vi "set_input_ref.vi"(8 "error in (no error)":errorcluster, 10 "input_ref":refnum<data-value>, 11 "input_poller in":refnum<class "input_poller.lvclass">) -> (0 "error out":errorcluster, 3 "input_poller out":refnum<class "input_poller.lvclass">)   [LabVIEW 2015, in "input_poller.lvclass"]
uses:
  input_poller.lvclass
  input.lvclass
  input_poller.lvclass/input_poller.ctl
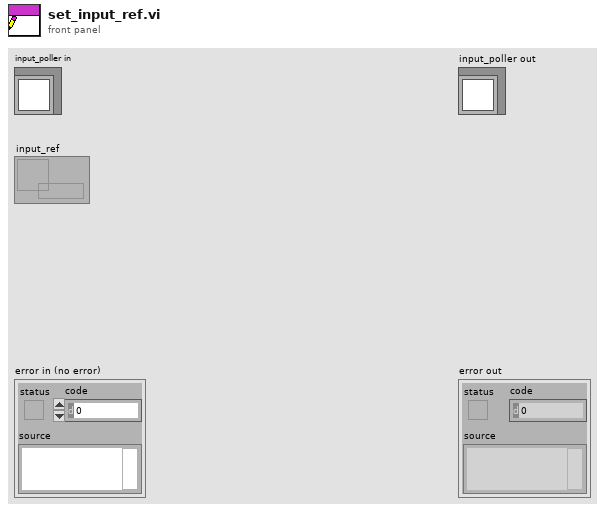
[diagram p1: front panel]
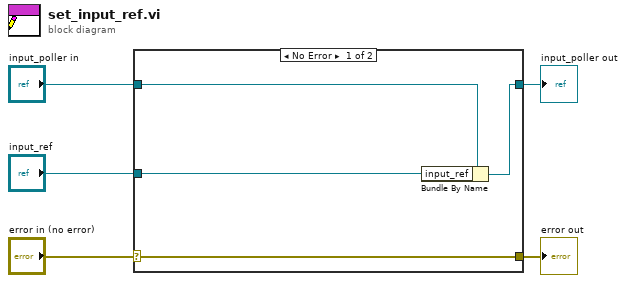
[diagram p0: block diagram]
diagram:
  n1 = case shown="No Error" "error in (no error)" {
    selector: "error in (no error)" -> [w9 w10]
    tunnel: [w9 w10] -> w4
    tunnel: [w7 w11] -> w2
    tunnel: "input_poller in" -> [w8 w11]
    tunnel: "input_ref" -> [w6 _]
    frame No Error {
      n2 = Bundle By Name(cluster=w8, "input_ref"=w6) -> (w7:refnum<class "input_poller.lvclass">)
    }
    frame Error {
    }
  }
  "error out" <- w4
  "input_poller out" <- w2
